vi "Store Data.vi"(4 "Time Array":string[](array[string]), 5 "Create Folder":bool, 6 "Date Array":string[](array[string]), 7 "Time Stamp":timestamp, 8 "Error In":errorcluster, 9 "S/N":string, 10 "Data Array":dbl[][](array[numeric]), 11 "Data Dir":path=path "C:/Test/LIDT/Data") -> (0 "Error Out":errorcluster, 3 "File Path Out":path)   [LabVIEW 2017]
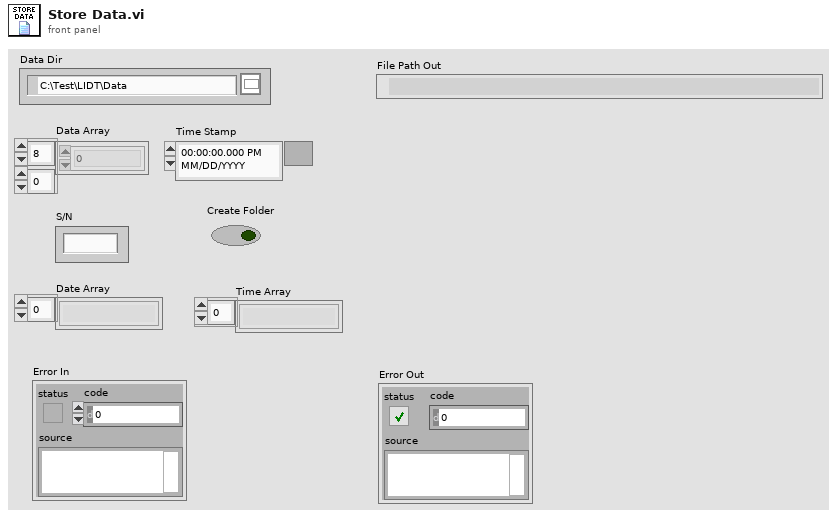
[diagram p1: front panel]
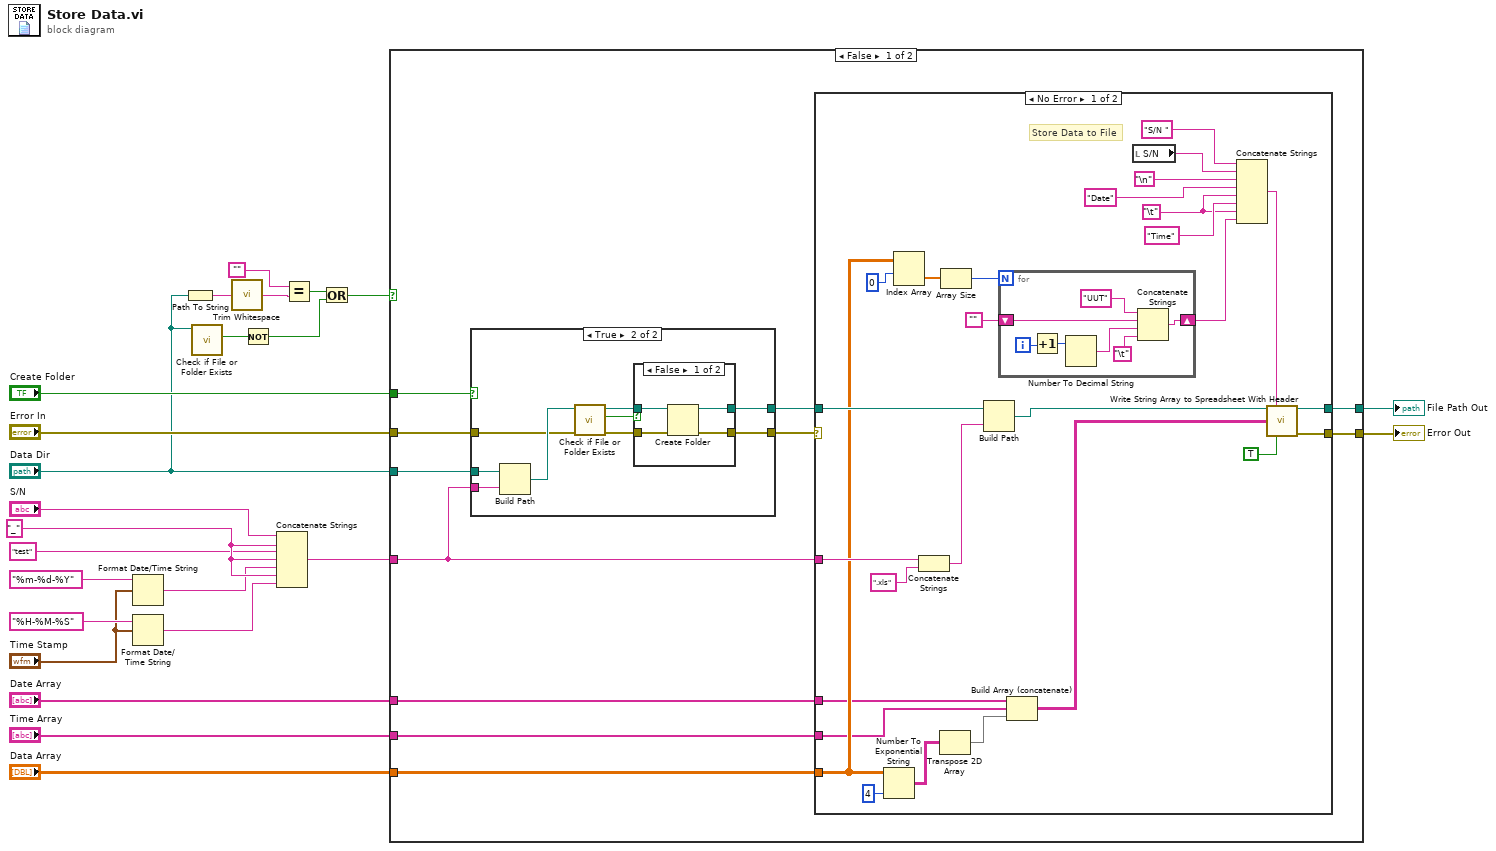
[diagram p0: block diagram]
diagram:
  w20 = "_" ("string")
  n1 = Format Date/Time String(time format string (%c)="%m-%d-%Y", seconds (now)="Time Stamp") -> (date/time string=w19:string)  [unwired: 1 in]
  n2 = Format Date/Time String(time format string (%c)="%H-%M-%S", seconds (now)="Time Stamp") -> (date/time string=w18:string)  [unwired: 1 in]
  n3 = Path To String(path="Data Dir") -> (string=w11:string)
  n4 = call <vilib>:"Check if File or Folder Exists.vi"("path"="Data Dir") -> ("file or folder exists?"=w7:bool)  [unwired: 8 in, 2 out]
  n5 = call <vilib>:"Trim Whitespace.vi"("string"=w11) -> ("trimmed string"=w9:string)  [unwired: 1 in]
  n6 = Not(x=w7) -> (.not. x?=w5:bool)
  n7 = Concatenate Strings("S/N", w20, "test" ("string"), w20, w19, w20, w18) -> (w24:string)
  n8 = Equal?(x="", y=w9) -> (x = y?=w6:bool)
  n9 = Or(x=w6, y=w5) -> (x .or. y?=w4:bool)
  n10 = case shown="False" w4 {
    tunnel: w24 -> [w28 _]
    tunnel: "Data Dir" -> [w35 w89]
    tunnel: "Error In" -> [w34 w90]
    tunnel: "Create Folder" -> [w33 _]
    tunnel: [w30 w89] -> w13
    tunnel: [w29 w90] -> w12
    tunnel: "Time Array" -> [w27 _]
    tunnel: "Data Array" -> [w26 _]
    tunnel: "Date Array" -> [w25 _]
    frame False {
      n11 = case shown="True" w33 {
        tunnel: w28 -> [_ w82]
        tunnel: [w73 w74] -> w32
        tunnel: w35 -> [w72 w81]
        tunnel: w34 -> [w73 w79]
        tunnel: [w72 w75] -> w31
        frame False {
        }
        frame True {
          n12 = Build Path(base path=w81, name or relative path=w82) -> (appended path=w80:path)
          n13 = call <vilib>:"Check if File or Folder Exists.vi"("error in (no error)"=w79, "path"=w80) -> ("error out"=w76:errorcluster, "file or folder exists?"=w78:bool, "dup path"=w77:path)  [unwired: 7 in]
          n14 = case shown="False" w78 {
            tunnel: w77 -> [w86 w88]
            tunnel: w76 -> [w85 w87]
            tunnel: [w84 w88] -> w75
            tunnel: [w83 w87] -> w74
            frame False {
              n15 = Create Folder(path (use dialog)=w86, error in=w85) -> (created path=w84:path, error out=w83:errorcluster)  [unwired: 1 in, 1 out]
            }
            frame True {
            }
          }
        }
      }
      n16 = case shown="No Error" w32 {
        selector: w32 -> [_ w70]
        tunnel: w31 -> [w62 w71]
        tunnel: [w54 w71] -> w30
        tunnel: [w53 w70] -> w29
        tunnel: w28 -> [w56 _]
        tunnel: w27 -> [w44 _]
        tunnel: w26 -> [w46 _]
        tunnel: w25 -> [w45 _]
        frame No Error {
          w37 = "\t"
          # "Store Data to File"
          n17 = Number To Exponential String(number=w46, precision (6)=i16 4) -> (E-format string=w40:string[][])  [unwired: 2 in]
          n18 = Index Array(array=w46, index (row)=0 ("disabled index (col)")) -> (element=w50:dbl[])  [unwired: 1 in]
          n19 = Concatenate Strings(w56, ".xls") -> (w60:string)
          n20 = Transpose 2D Array(2D array=w40) -> (transposed array=w39:string[][])
          n21 = Array Size(array=w50) -> (size(s)=w49:i32)
          n22 = Build Path(base path=w62, name or relative path=w60) -> (appended path=w55:path)
          n23 = for {
            N: w49 -> [_]
            shift-right: [w69] -> w36
            shift-left: "" -> [w65]
            i -> [w68]
            n24 = Increment(x=w68) -> (x+1=w67:i32)
            n25 = Number To Decimal String(number=w67) -> (decimal integer string=w64:string)  [unwired: 1 in]
            n26 = Concatenate Strings("UUT", w65, w64, "\t") -> (w69:string)
          }
          n27 = Build Array (concatenate)(w45, w44, w39) -> (w42:string[][])
          n28 = local read "S/N"() -> (w57:string)
          n29 = Concatenate Strings("S/N " ("time format string (%c)"), w57, "\n", "Date", w37, "Time" ("string"), w37, w36) -> (w43:string)
          n30 = call "Write String Array to Spreadsheet With Header.vi"("file path (dialog if empty)"=w55, "Header"=w43, "Data String Array"=w42, "transpose? (no:F)"=TRUE) -> ("new file path (Not A Path if cancelled)"=w54:path, "error out"=w53:errorcluster)  [unwired: 10 in]
        }
        frame Error {
        }
      }
    }
    frame True {
    }
  }
  "File Path Out" <- w13
  "Error Out" <- w12
